vi "PCRE Extract Content from HTML.vi"(11 "HTML String":string="\n") -> (3 "Content":string="3110178 AE Screenpop\r\n   #bodyblock {background:#FAF9F5; border:solid #000000; border-width:0 1px 0 1px;}\r\n   #ff_label { background:#FAF9F5; width:120px; text-align:left; margin-left: 50px; font-size:11px; padding:5px;}\r\n   #ff { background:#FAF9F5; width:150px; text-align:left; margin-left: 50px; font-size:11px; padding:5px;}\r\n   #links { background:#FAF9F5; width:480px; text-align:left; margin-left: 50px; font-size:11px; padding:5px;}\r\nGheorghe Dragan\r\nGheorghe Dragan (RO)\r\nService Level:\r\nBasic| No Contracts\r\n \r\n        \r\nStr. Abrud\r\nBUCURESTI,   011315 RO\r\n733 854148\r\ngdf.dragan@gmail.com\r\nContact #: 5089265\r\nTSR\r\nMircea Emil Stremtan\r\nDSM\r\nMircea Emil Stremtan\r\nASM\r\nAttila Péter\r\nRSM\r\nPaul Hoerner de Roithberg\r\nHome\r\nCall Logs\r\nSR #StatusSeverityDateService LevelOwnerProductSummary\r\n3110178IN WORKNot Evaluated18-JAN-2018Basic | No ContractsMihai DorneaMultifunctionDAQclearing tasks in MAX\r\nSR Open for: 4 Days, 3 Hours \r\n                Resolve/Escalate By:\r\n                Channel:\r\n            Problem Code:\r\n            Resolution Code:\r\n            SW Version:\r\n            O/S:\r\n            NI Driver:\r\n            Run HDD Diagnostic?\r\n            Branch SR:\r\n            LV NXG:\r\n PHONE        \r\nCustomer E-mail Interaction22-JAN-2018Mihai Dornea\r\nBuna ziua,\r\nAm sa va raspund la intrebari in ordinea in care au fost puse:\r\n- Aplicatia standalone va rula pe Windows 64 biti daca aceasta va fi configurata astfel si va arata intocmai precum va fi programata sa arate\r\n- Denumirea este LabVIEW Home Bundle\r\n- Pachetul contine applicatia de sine-statatoare LabVIEW Full Development System 2014 si 3 add-onuri pentru aceasta (tool-uri)\r\n- Programul este compatibil cu Windows 10 insa NI teoretic nu ofera support de dezvoltare pentru aceasta configuratie\r\n- Aici este discutabil in sensul urmator. Daca sunteti familiarizat cu programarea atunci singurele probleme ar fi partea de DAQmx (initializarea si folosirea propriu-zisa a modulului 6008) si partea de Interfata Grafica. Din fericire, comunitatea online este foarte mare si gasiti raspunsuri pentru orice intrebare legata de aceste parti. De asemenea exista si multe tutoriale on-line pentru a va familiariza cu mediul de programare.\r\n- Da, insa nu trebuie sa le cautati neaparat pe site-ul NI. LabVIEW vine cu o suita de exemple pentru cam orice tip de functie. In LabVIEW veti avea un buton Help in bara de activitati si un buton Find Examples in meniul de drop-down.\r\n- Da, care este chiar bogata din punct de vedere al continutului, de la operatii numerice simple la functii polinomiale complexe, interpolare si extrapolare, geometrie, probabilitati si statistica.\r\nDaca mai aveti intrebari aditionale nu ezitati sa ma contactati.\r\nCu respect,\r\nMihai Dornea\r\nNational Instruments\r\nApplications Engineering\r\nwww.ni.com/support\r\nCustomer E-mail Interaction22-JAN-2018Mihai Dornea\r\nBuna seara Domnule Dornea,\r\nInteleg ca LabView Full Development si Application Builder (pct.2 din mesaj) pot rezolva problema pe care v-am trimis-o atasat (flow-chart in 4 pasi).\r\n50 $ as putea duce, insa mai intai vreau sa stiu sigur niste aspecte:\r\n- as dori sa stiu sigur daca programul stand-alone final va arata pe ecranul PC exact asa cum am descris in flow-chart si va putea fi rulat pe orice PC care are instalat Windows 64 bit;\r\n- pe pagina de download pe care mi-ati indicat-o este denumirea LabView Bundle;corect? \r\n- programul contine de fapt 2 sub-programe, adica LabView propriu-zis si programul de convertire in stand-alone? sau este un program unic cu Application Builder sub forma de tool?\r\n- pe pagina de download se specifica ca acest program este compatibil cu Windows 10, insa NI \"nu suporta programul pe Windows 10\" ?\r\n- credeti ca ma pot descurca fara o scolarizare cat de cat?\r\n- exista postate pe site-urile NI niste exemple simple din care sa ma pot orienta?Daca da, atunci poate-mi trimteti niste link-uri.\r\n- programul LabView Full Development are si o biblioteca proprie de functii matematice ? \r\ncu multumiri pentru ajutor,\r\nDragan\r\nCustomer E-mail Interaction19-JAN-2018Mihai Dornea\r\nBuna ziua,\r\nIn cazul in care doriti sa realizati o aplicatie stand-alone, acest lucru este imposibil folosind o versiune Trial de LabVIEW, pentru aceasta fiind necesar modulul Application Builder, care costa destul de mult.\r\nAveti in schimb 2 variante pentru a putea realiza acest proiect.\r\n1. Va descarcati LabVIEW student edition care este gratuit pe o perioada mai lunga de timp, dar nu veti avea acces la Application Builder.\r\n2. https://store.digilentinc.com/labview-home-bundle/ Acesta este un pachet care contine LabVIEW Full Development si Application Builder, prin care puteti crea acea aplicatie standalone. Pachetul respectiv este doar 50 de dolari si obtineti si o licenta permanenta pe aceste software-uri.\r\nDaca mai aveti intrebari, va stau la dispozitie.\r\nO zi buna in continuare!\r\nCu respect,\r\nMihai Dornea\r\nNational Instruments\r\nApplications Engineering\r\nwww.ni.com/support\r\nCustomer E-mail Interaction19-JAN-2018Mihai Dornea\r\nSalut D-l Dornea,\r\nsi multumesc pt raspuns.Deocamdata o sa ma descurc in aceste conditii.\r\nCa sa achizitionez LabView este practic imposibil pentru ca nu-mi permit.Sunt pensionar cu un venit f limitat.\r\nTotusi as dori sa stiu daca se poate creia un program in LabView conform flow-chart atasat si care se poate ulterior converti intr-un program de sine-statator (standalone) ce poate fi rulat de oricine pe platforma Windows 64 bit dar fara ca utilizatorii sa aiba instalat LabView.\r\nMatlab, Maple si Wolfram (programe profesionale de matematica) au promis acest lucru, insa nu am reusit cu tot suportul tehnic din partea lor pe perioada cat am instalat de proba aceste programe (ultimele versiuni).\r\nCateva cuvinte despre programul atasat: este vorba de un test mental bazat pe masurarea unor perioade de timp de 5, 10, 15 si 20 secunde de 8 ori fiecare valoare fara ca persoana testata=care masoara sa vada valorile pe timpul masurarii.Va rezulta o matrice cu 4 coloane si 8 linii care urmeaza sa fie transferata in Excel pt a fi prelucrata.\r\nAcesta este si scopul pt care folosesc acum DAQ 6008.\r\nEste un fel de cronometru ceva mai sofisticat cu rezolutie mai buna de 0.001 s.\r\nToate bune,\r\nGheorghe DRAGAN\r\nCustomer E-mail Interaction18-JAN-2018\r\nBuna ziua,\r\nM-am documentat despre problema dumneavoastra si am discutat si cu colegii, iar concluzia este ca din nefericire nu se poate realiza ceea ce dumneavoastra doriti.\r\nProblema consta in faptul ca NI Measurement and Automation Explorer este un program destul de limitat in ceea ce consta in \"programarea\" masuratorilor, in sensul in care este mai mult folosit pentru testare sau pentru configurarea unor setari pentru a fi folosite in LabVIEW.\r\nDin acest motiv, task-urile in sine nu au optiuni avansate de modelare a datelor, acest lucru trebuie programat in LabVIEW, deoarece LabVIEW este mediul in care aceste masuratori sunt puse cu adevarat in valoare.\r\nDaca mai aveti intrebari, va stau la dispozitie.\r\nVa multumesc si o zi buna in continuare!\r\nCu respect,\r\nMihai Dornea\r\nNational Instruments\r\nApplications Engineeringwww.ni.com/support\r\nDisplay more service requests for this contact")   [LabVIEW 2017]
uses:
  <vilib>/regexp/Match Regular Expression.xnode
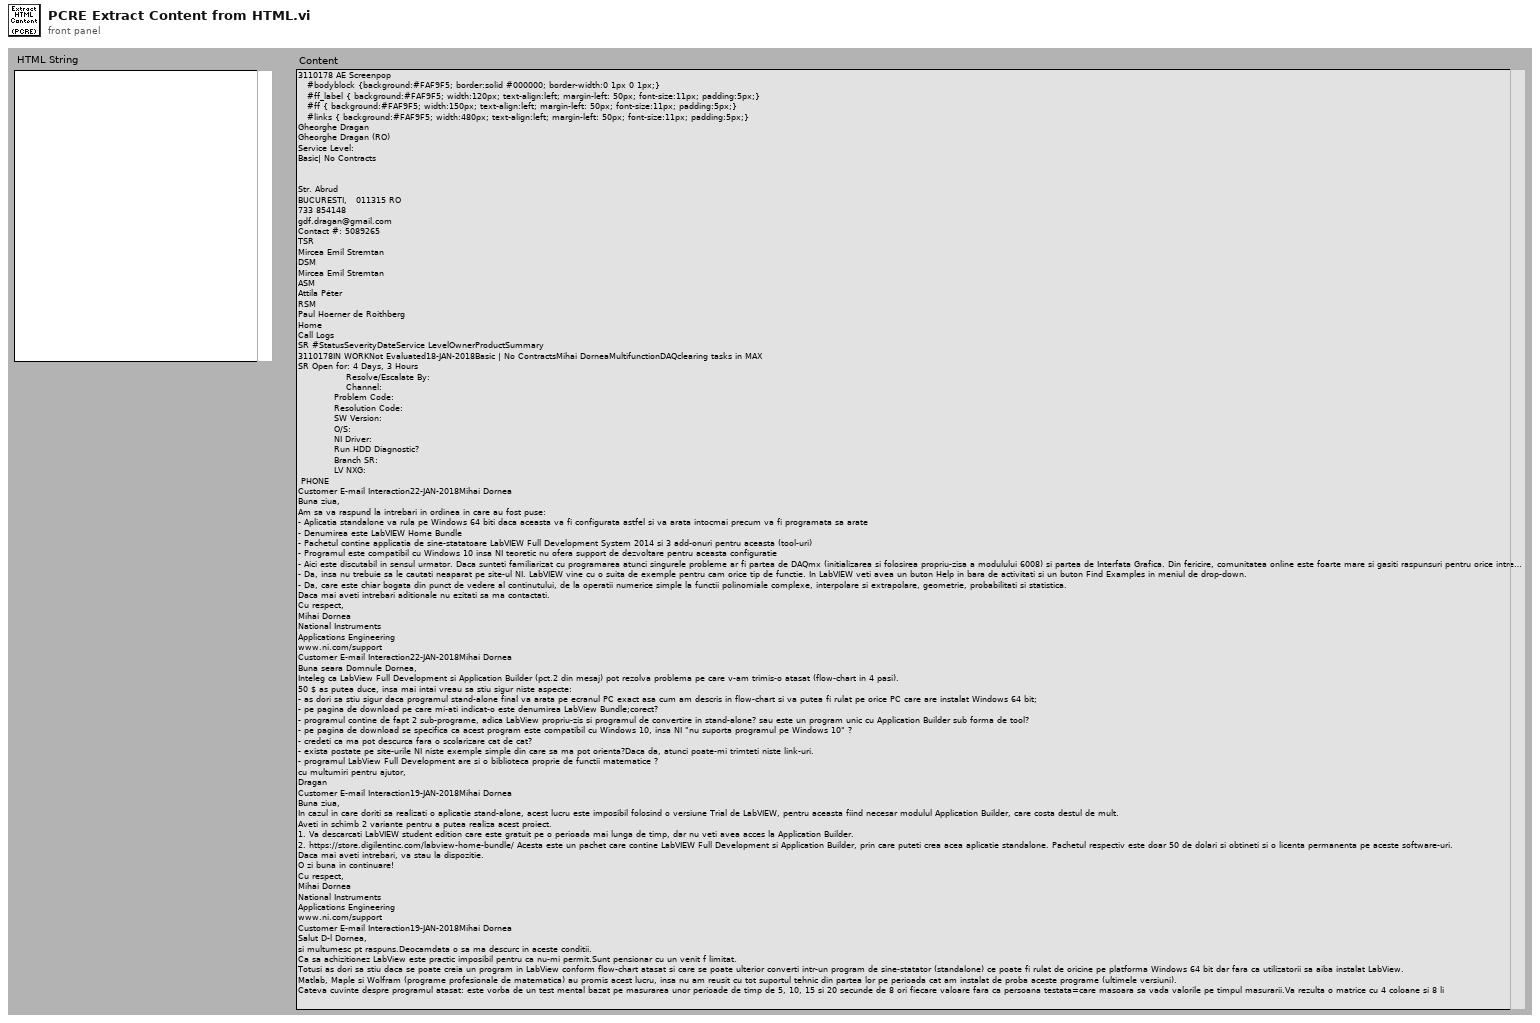
[diagram p1: front panel]
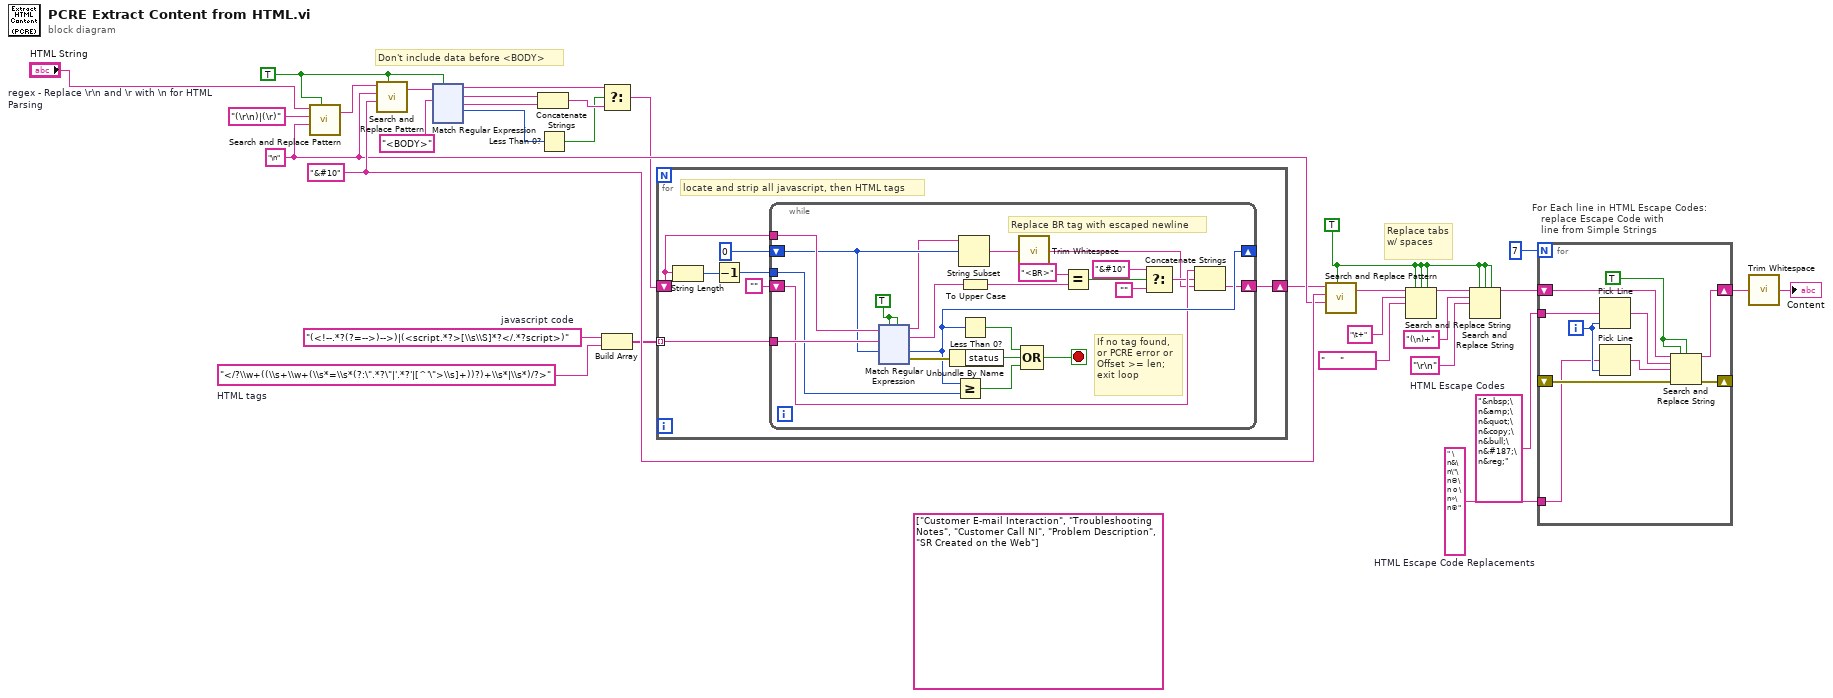
[diagram p0: block diagram]
diagram:
  (unwired) string[] ["Customer E-mail Interaction", "Troubleshooting Notes", "Customer Call NI", "Problem Description", "SR Created on the Web"]
  w9 = "(<!--.*?(?=-->)-->)|(<script.*?>[\\s\\S]*?</.*?script>)"  # javascript code
  w20 = " \n&\n\"\n©\n o \n»\n®"  # HTML Escape Code Replacements
  w22 = "&nbsp;\n&amp;\n&quot;\n&copy;\n&bull;\n&#187;\n&reg;"  # HTML Escape Codes
  w1 = TRUE ("replace all? (F)")
  w2 = TRUE ("replace all? (F)")
  w23 = "\n" ("replace string (\"\")")
  w25 = "(\r\n)|(\r)"  # regex - Replace \r\n and \r with \n for HTML Parsing
  w24 = "&#10" ("replace string (\"\")")
  w16 = "</?\\w+((\\s+\\w+(\\s*=\\s*(?:\".*?\"|'.*?'|[^'\">\\s]+))?)+\\s*|\\s*)/?>"  # HTML tags
  # "Don't include data before <BODY>"
  # "Replace tabs w/ spaces"
  n1 = call <vilib>:"Search and Replace Pattern.vi"("string"="HTML String", "regular expression (\"\")"=w25, "replace string (\"\")"=w23, "replace all? (F)"=w2) -> ("result string"=w6:string)  [unwired: 2 out]
  n2 = call <vilib>:"Search and Replace Pattern.vi"("string"=w6, "regular expression (\"\")"=w23, "replace string (\"\")"=w24, "replace all? (F)"=w2) -> ("result string"=w8:string)  [unwired: 2 out]
  n3 = xnode "Match Regular Expression"("input string"=w8, "regular expression"="<BODY>", "ignore case? (F)"=w2) -> ("before match"=w26:string, "whole match"=w29:string, "after match"=w28:string, "offset past match"=w30:i32)  [unwired: 2 in, 2 out]
  n4 = Concatenate Strings(w29, w28) -> (w32:string)
  n5 = Less Than 0?(x=w30) -> (x < 0?=w31:bool)
  n6 = Select(t=w26, s=w31, f=w32) -> (s? t:f=w15:string)
  n7 = Build Array(w9, w16) -> (w14:string[])
  n8 = for {
    shift-right: [w35] -> w17
    shift-left: w15 -> [w34]
    tunnel: w14 -> [w33] mode=indexing
    # "locate and strip all javascript, then HTML tags"
    n9 = String Length(string=w34) -> (length=w39:i32)
    n10 = Decrement(x=w39) -> (x-1=w38:i32)
    n11 = while {
      shift-right: [w45] -> w35
      shift-left: "" -> [w47]
      shift-right: [w53] -> _
      shift-left: 0 ("offset (0)") -> [w52]
      tunnel: w34 -> [w62]
      tunnel: w33 -> [w61]
      tunnel: w38 -> [w55]
      stop <- w56 stop-if-true
      w43 = TRUE ("ignore case? (F)")
      # "Replace BR tag with escaped newline"
      # "If no tag found,\nor PCRE error or\nOffset >= len;\nexit loop"
      n12 = xnode "Match Regular Expression"("input string"=w62, "regular expression"=w61, "offset (0)"=w52, "ignore case? (F)"=w43, "multiline? (F)"=w43) -> ("before match"=w44:string, "whole match"=w49:string, "offset past match"=w53:i32, "error out"=w60:errorcluster)  [unwired: 1 in, 1 out]
      n13 = Unbundle By Name(w60) -> ("status"=w58:bool)
      n14 = Greater Or Equal?(x=w53, y=w55) -> (x >= y?=w57:bool)
      n15 = String Subset(string=w44, offset (0)=w52) -> (substring=w54:string)  [unwired: 1 out]
      n16 = To Upper Case(1:w49) -> (0:w41:string)
      n17 = Less Than 0?(x=w53) -> (x < 0?=w59:bool)
      n18 = call <vilib>:"Trim Whitespace.vi"("string"=w54) -> ("trimmed string"=w42:string)  [unwired: 1 in]
      n19 = Compound Arithmetic op=OR(w59, w58, w57) -> (w56:bool)
      n20 = Equal?(x="<BR>", y=w41) -> (x = y?=w50:bool)
      n21 = Select(t="&#10", s=w50, f="") -> (s? t:f=w46:string)
      n22 = Concatenate Strings(w47, w46, w42) -> (w45:string)
    }
  }
  n23 = call <vilib>:"Search and Replace Pattern.vi"("string"=w17, "regular expression (\"\")"=w24, "replace string (\"\")"=w23, "replace all? (F)"=w1) -> ("result string"=w4:string)  [unwired: 2 out]
  n24 = Search and Replace String(replace all?=w1, case sensitive?=w1, multiline?=w1, input string=w4, search string="\t+" ("replace string (\"\")"), replace string="     " ("search string")) -> (result string=w3:string)  [unwired: 1 in, 4 out]
  n25 = Search and Replace String(replace all?=w1, case sensitive?=w1, multiline?=w1, input string=w3, search string="(\n)+", replace string="\r\n" ("search string")) -> (result string=w5:string)  [unwired: 1 in, 4 out]
  n26 = for "For Each line in HTML Escape Codes:\n   replace Escape Code with \n   line from Simple Strings" {
    N: 7 -> [_]
    shift-right: [w185] -> w19
    shift-left: w5 -> [w184]
    shift-right: [w179] -> _
    shift-left: _ -> [w180]
    tunnel: w22 -> [w178]
    tunnel: w20 -> [w177]
    i -> [w181]
    w186 = TRUE ("replace all? (F)")
    n27 = Pick Line(multi-line string=w178, line index=w181) -> (output string=w183:string)  [unwired: 1 out]
    n28 = Pick Line(multi-line string=w177, line index=w181) -> (output string=w182:string)  [unwired: 1 out]
    n29 = Search and Replace String(replace all?=w186, case sensitive?=w186, input string=w184, search string=w183, replace string=w182, error in=w180) -> (result string=w185:string, error out=w179:errorcluster)  [unwired: 1 in, 3 out]
  }
  n30 = call <vilib>:"Trim Whitespace.vi"("string"=w19) -> ("trimmed string"=→"Content":string)  [unwired: 1 in]
